vi "SecondaryRobotFunctions.vi"(8 "Secondary Joystick Values":dbl[](array[numeric]), 9 "ADIS Gyro Values":T1 {"IMU Data Out"."X Accel (g)" format="%#_3g"; "IMU Data Out"."Y Accel (g)" format="%#_3g"; "IMU Data Out"."Z Accel (g)" format="%#_3g"}, 10 "Drive Joystick Buttons":bool[](array[boolean]), 11 "Secondary Joystick Buttons":bool[](array[boolean])) -> ()   [LabVIEW 2018]
uses:
  ADIS Gyro Values.ctl
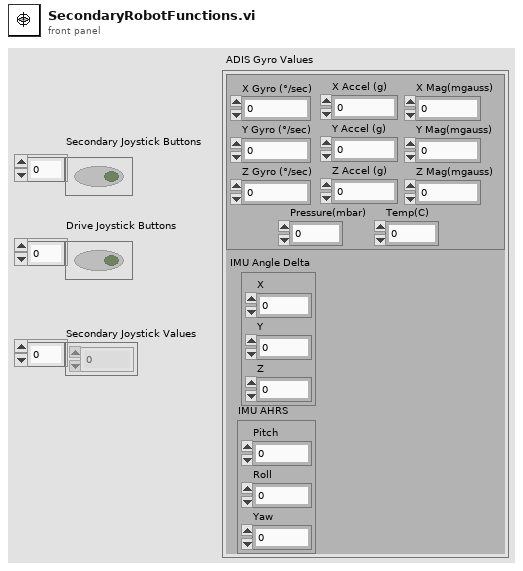
[diagram p1: front panel]
types:
  T1 = typedef "ADIS Gyro Values.ctl" = cluster{"IMU Data Out":cluster{"X Gyro (°/sec)":dbl, "Y Gyro (°/sec)":dbl, "Z Gyro (°/sec)":dbl, "X Accel (g)":dbl, "Y Accel (g)":dbl, "Z Accel (g)":dbl, "X Mag(mgauss)":dbl, "Y Mag(mgauss)":dbl, "Z Mag(mgauss)":dbl, "Pressure(mbar)":dbl, "Temp(C)":dbl}, "IMU Angle Delta":cluster{"X":dbl, "Y":dbl, "Z":dbl}, "IMU AHRS":cluster{"Pitch":dbl, "Roll":dbl, "Yaw":dbl}}
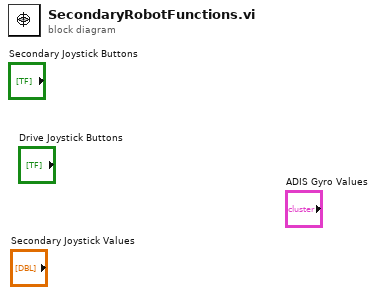
[diagram p0: block diagram]
diagram:
